vi "Importance of Type Definitions.vi"() -> ()   [LabVIEW 2020]
panel:
  in  "Title":T1(ring)
  out "Employee Record Out":T2={"First Name"="Jennifer", "Preferred Name"="Jenny", "Surname"="Swift", "Department"=enum."Finance", "Employment Status"=enum."Part Time", "Start Date"=timestamp(3565024425.501588 s since 1904-01-01), "Normal Working Location"=enum."Working in Office"} {"Start Date" format="%<%x %.3X>T"}
  in  "Employee Record In":T2={"First Name"="Jennifer", "Preferred Name"="Jenny", "Surname"="Swift", "Department"=enum."Finance", "Employment Status"=enum."Part Time", "Start Date"=timestamp(3565024425.501588 s since 1904-01-01), "Normal Working Location"=enum."Working in Office"} {"Start Date" format="%<%x %.3X>T"}
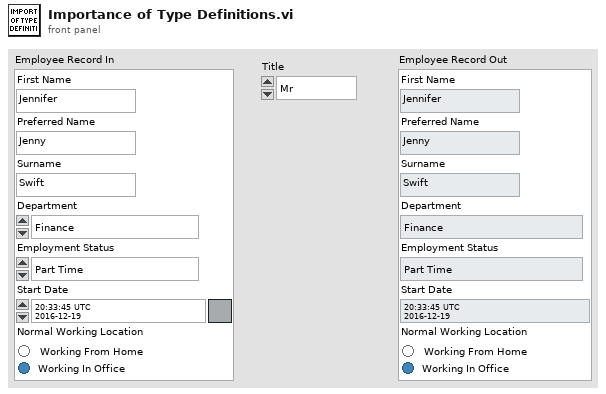
[diagram p1: front panel]
types:
  T1 = enum16{"Mr", "Mrs", "Ms", "Mx", "Miss", "Sir", "Dame", "Other"}
  T2 = cluster{"First Name":string, "Preferred Name":string, "Surname":string, "Department":enum16{"Research and Development", "Technical Support", "Sales", "Management", "Finance", "Other"}, "Employment Status":enum16{"Full Time", "Part Time", "No Longer Employed", "Probation", "Other"}, "Start Date":timestamp, "Normal Working Location":enum32{"Working From Home", "Working in Office"}}
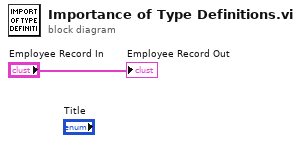
[diagram p0: block diagram]
diagram:
  "Employee Record Out" <- "Employee Record In"
